vi "ConvertBanksToScanList.vi"(7 "Slot":T1, 8 "Bank D Channel Enabled":bool[](array[boolean]), 9 "Bank C Channel Enabled":bool[](array[boolean]), 10 "Bank B Channel Enabled":bool[](array[boolean])=[FALSE, FALSE, FALSE, FALSE, FALSE, FALSE, FALSE, FALSE, FALSE, FALSE], 11 "Bank A Channel Enabled":bool[](array[boolean])) -> (3 "Scan List":string)   [LabVIEW 2012]
uses:
  driver/Public/Controls/Slot.ctl
  driver/Keithley-7001.lvlib
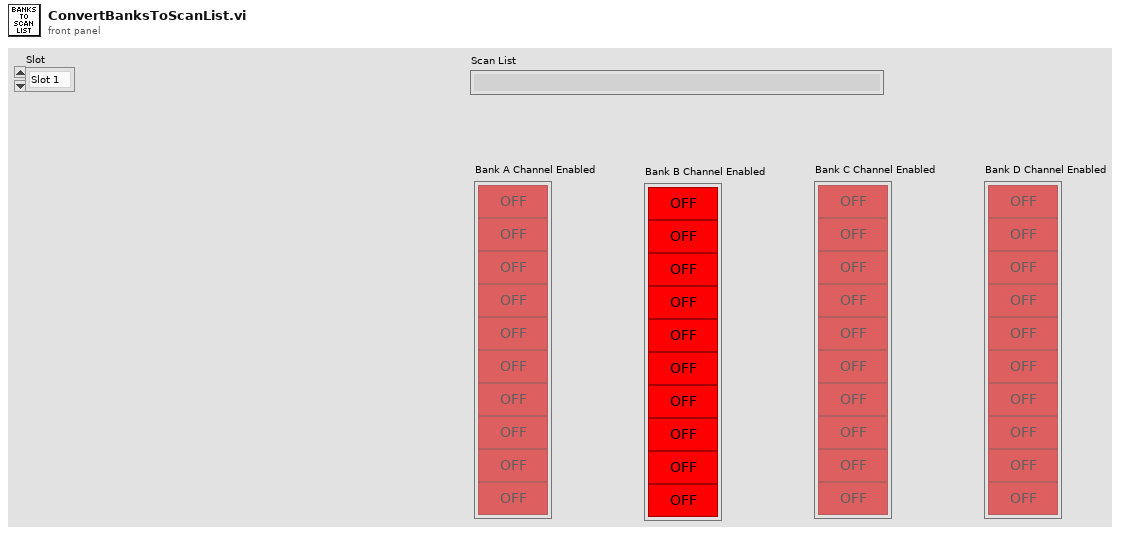
[diagram p1: front panel]
types:
  T1 = typedef "Keithley-7001.lvlib/Slot.ctl" = enum16{"Slot 1", "Slot 2"}
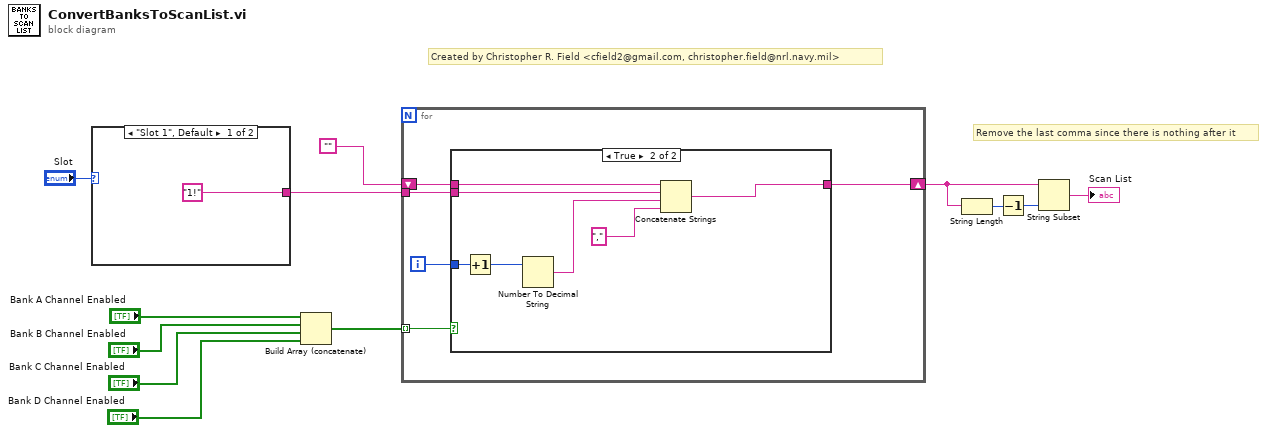
[diagram p0: block diagram]
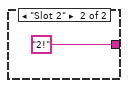
[diagram p2: hidden frame]
diagram:
  # "Created by Christopher R. Field <cfield2@gmail.com, christopher.field@nrl.navy.mil>"
  # "Remove the last comma since there is nothing after it"
  n1 = case shown="\"Slot 1\", Default" "Slot" {
    tunnel: ["1!" "2!"] -> w10
    frame "Slot 1", Default {
    }
    frame "Slot 2" {
    }
  }
  n2 = Build Array (concatenate)("Bank A Channel Enabled", "Bank B Channel Enabled", "Bank C Channel Enabled", "Bank D Channel Enabled") -> (w12:bool[])
  n3 = for {
    tunnel: w12 -> [w15] mode=indexing
    shift-right: [w17] -> w9
    shift-left: "" -> [w19]
    tunnel: w10 -> [w16]
    i -> [w18]
    n4 = case shown="True" w15 {
      tunnel: w19 -> [w20 w27]
      tunnel: w18 -> [_ w26]
      tunnel: [w20 w24] -> w17
      tunnel: w16 -> [_ w21]
      frame False {
      }
      frame True {
        n5 = Increment(x=w26) -> (x+1=w25:i32)
        n6 = Number To Decimal String(number=w25) -> (decimal integer string=w22:string)  [unwired: 1 in]
        n7 = Concatenate Strings(w27, w21, w22, "," ("string")) -> (w24:string)
      }
    }
  }
  n8 = String Length(string=w9) -> (length=w8:i32)
  n9 = Decrement(x=w8) -> (x-1=w7:i32)
  n10 = String Subset(string=w9, length (rest)=w7) -> (substring=→"Scan List":string)  [unwired: 1 in]
